vi "Get Error Info.vi"(11 "Base Actor in":refnum<class "Base Actor.lvclass">) -> (2 "Error Info":T1)   [LabVIEW 2020, in "jettl.lvlib" / "Actor.lvlib" / "Base Actor.lvclass"]
uses:
  Base Actor.lvclass
  Error Info.ctl
  Base Actor.lvclass/Base Actor.ctl
  Actor.lvlib
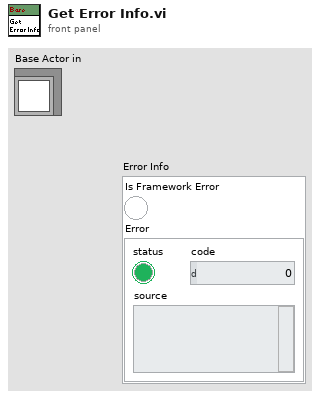
[diagram p1: front panel]
types:
  T1 = typedef "jettl.lvlib/Actor.lvlib/Error Info.ctl" = cluster{"Is Framework Error":bool, "Error":errorcluster}
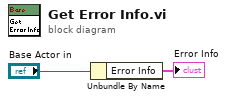
[diagram p0: block diagram]
diagram:
  n1 = Unbundle By Name("Base Actor in") -> ("Error Info"=→"Error Info":T1)
